vi "Scale_Sensor_Data.vi"(8 "Gravitation-Constant":dbl=9.81, 10 "Dataset":i16, 11 "Measurement Type":u16 format="%x") -> (0 "Sensor":string, 1 "Unit":string, 2 "Scaled Measurement":dbl, 3 "Alarm Array":bool[](array[boolean]))   [LabVIEW 2013]
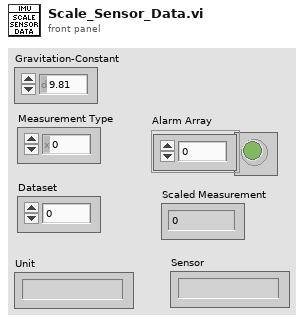
[diagram p1: front panel]
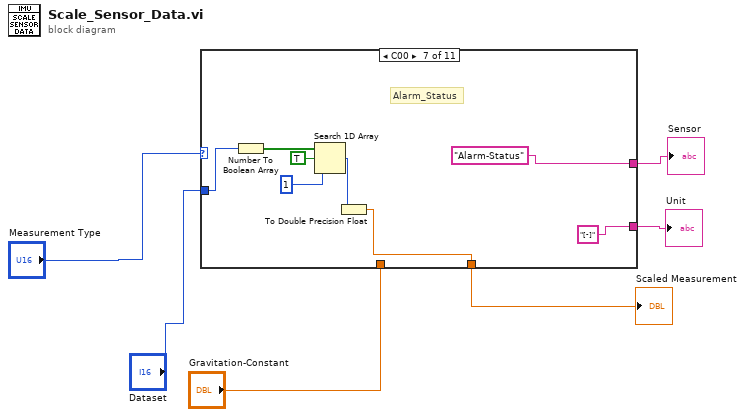
[diagram p0: block diagram]
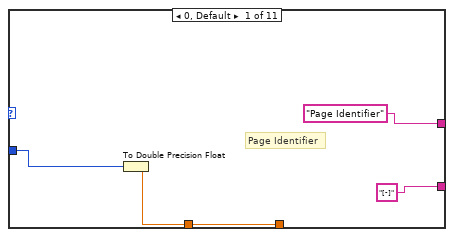
[diagram p2: hidden frame]
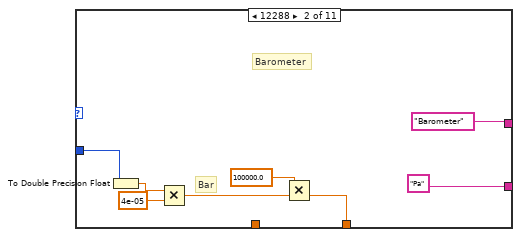
[diagram p3: hidden frame]
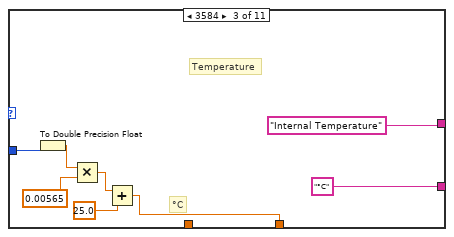
[diagram p4: hidden frame]
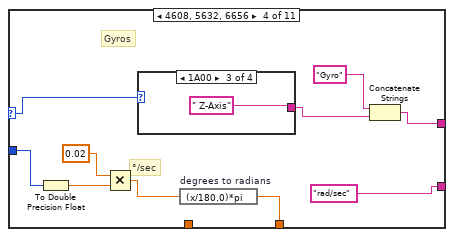
[diagram p5: hidden frame]
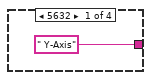
[diagram p6: hidden frame]
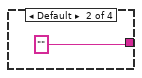
[diagram p7: hidden frame]
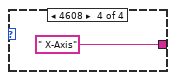
[diagram p8: hidden frame]
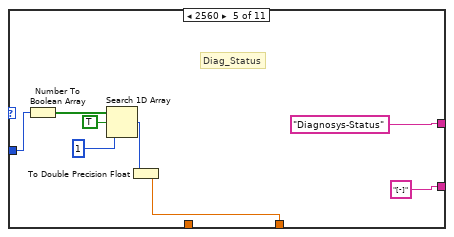
[diagram p9: hidden frame]
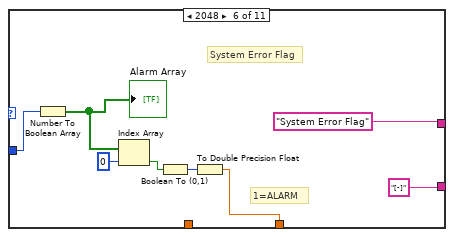
[diagram p10: hidden frame]
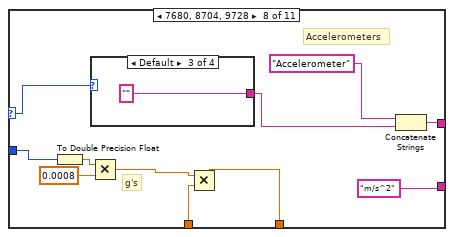
[diagram p11: hidden frame]
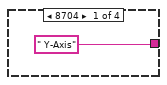
[diagram p12: hidden frame]
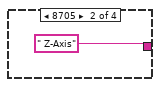
[diagram p13: hidden frame]
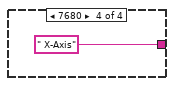
[diagram p14: hidden frame]
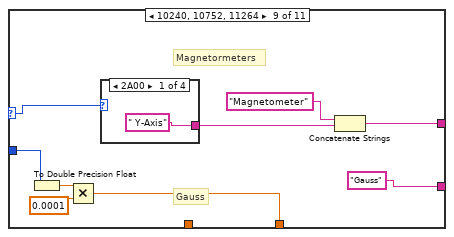
[diagram p15: hidden frame]
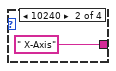
[diagram p16: hidden frame]
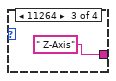
[diagram p17: hidden frame]
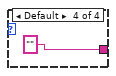
[diagram p18: hidden frame]
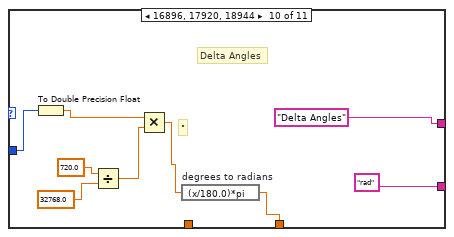
[diagram p19: hidden frame]
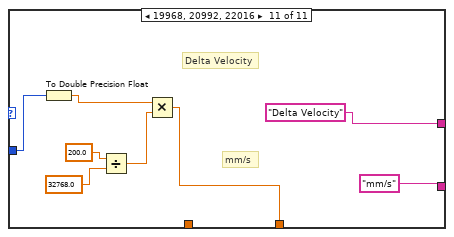
[diagram p20: hidden frame]
diagram:
  n1 = case shown="C00" "Measurement Type" {
    selector: "Measurement Type" -> [_ _ _ w32 _ _ _ w71 w80 _ _]
    tunnel: "Dataset" -> [w9 w18 w26 w35 w43 w51 w59 w75 w88 w97 w105]
    tunnel: [w10 w12 w22 w27 w44 w52 w60 w67 w86 w93 w104] -> w6
    tunnel: ["[-]" "Pa" "°C" "rad/sec" "[-]" "[-]" "[-]" "m/s^2" "Gauss" "rad" "mm/s"] -> w3
    tunnel: ["Page Identifier" "Barometer" "Internal Temperature" w29 "Diagnosys-Status" "System Error Flag" "Alarm-Status" w70 w81 "Delta Angles" "Delta Velocity"] -> w2
    tunnel: "Gravitation-Constant" -> [_ _ _ _ _ _ _ w65 _ _ _]
    frame 0, Default {
      # "Page Identifier"
      n2 = To Double Precision Float(number=w9) -> (double precision float=w10:dbl)
    }
    frame 12288 {
      # "Barometer"
      # "Bar"
      n3 = To Double Precision Float(number=w18) -> (double precision float=w17:dbl)
      n4 = Multiply(x=w17, y=4e-05) -> (x*y=w15:dbl)
      n5 = Multiply(x=100000.0, y=w15) -> (x*y=w12:dbl)
    }
    frame 3584 {
      # "°C"
      # "Temperature"
      n6 = To Double Precision Float(number=w26) -> (double precision float=w25:dbl)
      n7 = Multiply(x=w25, y=0.00565) -> (x*y=w23:dbl)
      n8 = Add(x=w23, y=25.0) -> (x+y=w22:dbl)
    }
    frame 4608, 5632, 6656 {
      # "Gyros"
      # "°/sec"
      n9 = To Double Precision Float(number=w35) -> (double precision float=w34:dbl)
      n10 = Multiply(x=0.02 ("y"), y=w34) -> (x*y=w28:dbl)
      n11 = case shown="1A00" w32 {
        tunnel: [" Y-Axis" "" " Z-Axis" " X-Axis"] -> w30
        frame 5632 {
        }
        frame Default {
        }
        frame 6656 {
        }
        frame 4608 {
        }
      }
      n12 = expression code="(x/180.0)*pi" "degrees to radians"(w28) -> (w27:dbl)
      n13 = Concatenate Strings("Gyro", w30) -> (w29:string)
    }
    frame 2560 {
      # "Diag_Status"
      n14 = Number To Boolean Array(number=w43) -> (Boolean array=w48:bool[])
      n15 = Search 1D Array(1D array=w48, element=TRUE, start index (0)=1) -> (index of element=w45:i32)
      n16 = To Double Precision Float(number=w45) -> (double precision float=w44:dbl)
    }
    frame 2048 {
      # "System Error Flag"
      # "1=ALARM"
      n17 = Number To Boolean Array(number=w51) -> (Boolean array=w56:bool[])
      "Alarm Array" <- w56
      n18 = Index Array(array=w56, index=0) -> (element=w54:bool)
      n19 = Boolean To (0,1)(Boolean=w54) -> (0, 1=w53:i16)
      n20 = To Double Precision Float(number=w53) -> (double precision float=w52:dbl)
    }
    frame 3072 {
      # "Alarm_Status"
      n21 = Number To Boolean Array(number=w59) -> (Boolean array=w64:bool[])
      n22 = Search 1D Array(1D array=w64, element=TRUE, start index (0)=1) -> (index of element=w61:i32)
      n23 = To Double Precision Float(number=w61) -> (double precision float=w60:dbl)
    }
    frame 7680, 8704, 9728 {
      # "Accelerometers"
      # "g's"
      n24 = To Double Precision Float(number=w75) -> (double precision float=w74:dbl)
      n25 = Multiply(x=w74, y=0.0008) -> (x*y=w66:dbl)
      n26 = case shown="Default" w71 {
        tunnel: [" Y-Axis" " Z-Axis" "" " X-Axis"] -> w68
        frame 8704 {
        }
        frame 8705 {
        }
        frame Default {
        }
        frame 7680 {
        }
      }
      n27 = Multiply(x=w66, y=w65) -> (x*y=w67:dbl)
      n28 = Concatenate Strings("Accelerometer", w68) -> (w70:string)
    }
    frame 10240, 10752, 11264 {
      # "Gauss"
      # "Magnetormeters"
      n29 = To Double Precision Float(number=w88) -> (double precision float=w87:dbl)
      n30 = Multiply(x=w87, y=0.0001) -> (x*y=w86:dbl)
      n31 = case shown="2A00" w80 {
        tunnel: [" Y-Axis" " X-Axis" " Z-Axis" ""] -> w82
        frame 10752 {
        }
        frame 10240 {
        }
        frame 11264 {
        }
        frame Default {
        }
      }
      n32 = Concatenate Strings("Magnetometer", w82) -> (w81:string)
    }
    frame 16896, 17920, 18944 {
      # "°"
      # "Delta Angles"
      n33 = To Double Precision Float(number=w97) -> (double precision float=w101:dbl)
      n34 = Divide(x=720.0, y=32768.0) -> (x/y=w98:dbl)
      n35 = Multiply(x=w101, y=w98) -> (x*y=w94:dbl)
      n36 = expression code="(x/180.0)*pi" "degrees to radians"(w94) -> (w93:dbl)
    }
    frame 19968, 20992, 22016 {
      # "Delta Velocity"
      # "mm/s"
      n37 = To Double Precision Float(number=w105) -> (double precision float=w109:dbl)
      n38 = Divide(x=200.0, y=32768.0) -> (x/y=w106:dbl)
      n39 = Multiply(x=w109, y=w106) -> (x*y=w104:dbl)
    }
  }
  "Scaled Measurement" <- w6
  "Unit" <- w3
  "Sensor" <- w2
